vi "SetUserLevel.vi"(0 "reference in":refnum<class "UI Manager Proxy.lvclass">, 2 "UserLevel":T1, 5 "Error In":errorcluster) -> (14 "reference out":refnum<class "UI Manager Proxy.lvclass">, 19 "Error Out":errorcluster)   [LabVIEW 2024, in "UI Manager Proxy.lvclass"]
uses:
  UI Manager Proxy.lvclass
  UI Manager Proxy.lvclass/UI Manager Proxy.ctl
  UserLevel.ctl
panel:
  # "Connector Pane"
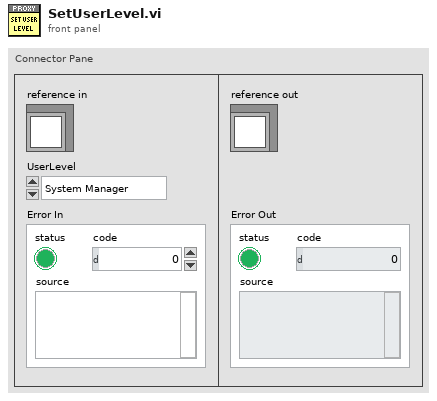
[diagram p1: front panel]
types:
  T1 = typedef "UserLevel.ctl" = enum16{"System Manager", "Admin", "Operator"}
  T2 = typedef "UI Manager Proxy.lvclass/ObjectAttributes.ctl" = cluster{"UI Manager":refnum<class "UI Manager.lvclass">, "UserLevel":T1}
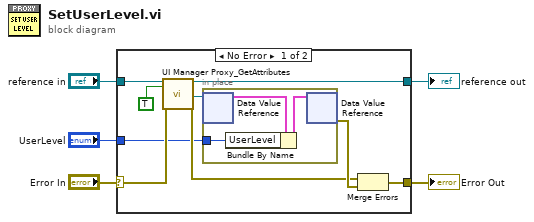
[diagram p0: block diagram]
diagram:
  n1 = case shown="No Error" "Error In" {
    selector: "Error In" -> [w12 w19]
    tunnel: [w7 w19] -> w4
    tunnel: [w13 w18] -> w2
    tunnel: "reference in" -> [w14 w18]
    tunnel: "UserLevel" -> [w6 _]
    frame No Error {
      n2 = call "UI Manager Proxy_GetAttributes.vi"("reference in"=w14, "OnlyGetDvrReference(False)"=TRUE, "Error In"=w12) -> ("reference out"=w13:refnum<class "UI Manager Proxy.lvclass">, "DataRef"=w9:refnum<data-value>, "Error Out"=w8:errorcluster)  [unwired: 13 in, 1 out]
      n3 = in-place {
        in-place-border: w6 -> [w15]
        n4 = in-place-dvr #1(w9) -> (w17:T2)  [unwired: 1 out]
        n5 = Bundle By Name(cluster=w17, "UserLevel"=w15) -> (w16:T2)
        n6 = in-place-dvr #1(w16) -> (w10:errorcluster)  [unwired: 1 out]
      }
      n7 = Merge Errors(w8, w10) -> (w7:errorcluster)
    }
    frame Error {
    }
  }
  "Error Out" <- w4
  "reference out" <- w2
